vi "COMI Get Resources.vi"(5 "nNumMemPorts":i32, 6 "pdwMemPorts":u32, 7 "nNumPorts":i32, 9 "pdwIoPorts":u32, 10 "pdwIntVect":u32, 11 "hDevice":u32) -> (1 "pdwIoPorts out":u32, 2 "pdwIntVect out":u32, 3 "hDevice out":u32, 4 "pdwMemPorts out":u32)   [LabVIEW 2017, in "Comidll.lvlib"]
doc: "void (COMI_GetResources) (HANDLE hDevice, unsigned long *pdwIntVect, unsigned long *pdwIoPorts,\n int nNumPorts, unsigned long *pdwMemPorts, int nNumMemPorts);"
uses:
  <userlib>/Comidll/Comidll.lvlib
  <userlib>/Comidll/Comidll.dll
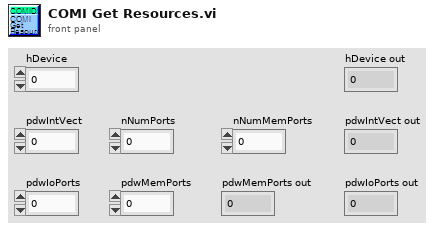
[diagram p1: front panel]
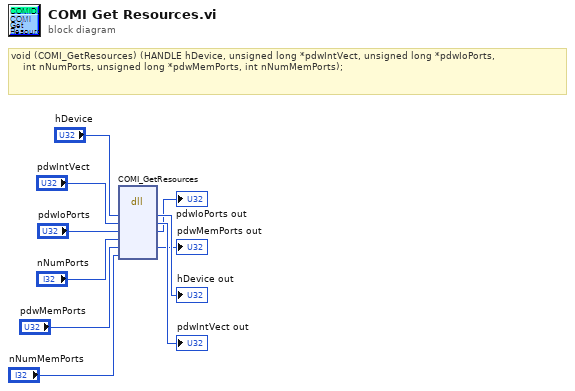
[diagram p0: block diagram]
diagram:
  # "void\t(COMI_GetResources) (HANDLE hDevice, unsigned long *pdwIntVect, unsigned long *pdwIoPorts,\n\t\t\t int nNumPorts, unsigned long *pdwMemPorts, int nNumMemPorts);"
  n1 = dll-call lib="C:/Program Files/National Instruments/LabVIEW 2017/user.lib/Comidll/Comidll.*" fn="COMI_GetResources"("hDevice"="hDevice", "pdwIntVect"="pdwIntVect", "pdwIoPorts"="pdwIoPorts", "nNumPorts"="nNumPorts", "pdwMemPorts"="pdwMemPorts", "nNumMemPorts"="nNumMemPorts") -> ("hDevice"=→"hDevice out":u32, "pdwIntVect"=→"pdwIntVect out":u32, "pdwIoPorts"=→"pdwIoPorts out":u32, "pdwMemPorts"=→"pdwMemPorts out":u32)  [unwired: 6 in, 2 out]
